vi "Gunsim Simulate.vi"(1 "Robot Constants":T4={"Distance from Pivot Point to Drive Mount(in)"=2.0, "Distance from Pivot Point to Arm Mount(in)"=2.0, "Distance from Pivot Point to Launcher(in)"=2.0, "Distance from Pivot Point to Camera(in)"=2.0, "WheelEncoder Ticks/Revolution"=2.0, "Wheel Radius"=2.0, "Triangle Angle(degrees)"=2.0, "Minimum LA Distance(inches)"=2.0, "LA Distance/Tick(inches)"=2.0}, 2 "cluster in":T3, 3 "Other Constants":T2={"Ball Diameter(in)"=10.0, "Air Density(g/in^3)"=0.02, "Drag coefficient"=0.5, "Ball Mass(g)"=300.0, "gravity(in/s^2)"=-386.09, "Minimum Goal Height(in)"=90.0, "Maximum Goal Height(in)"=104.0}, 4 "Parameters":T1) -> (0 "Range":T5)   [LabVIEW 2015]
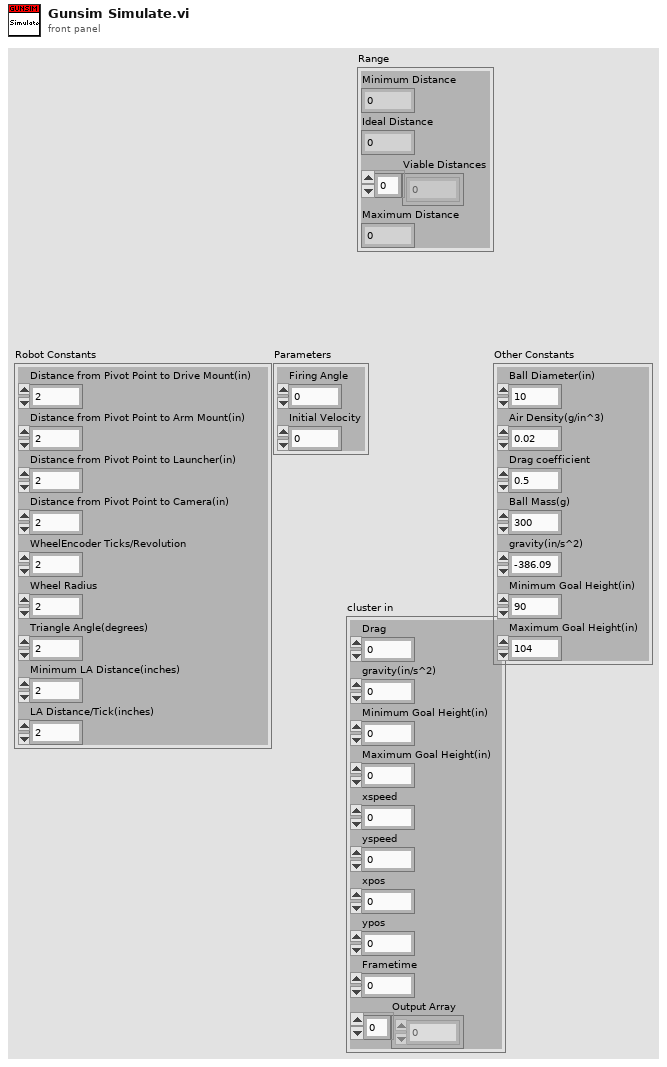
[diagram p1: front panel]
types:
  T1 = cluster{"Firing Angle":dbl, "Initial Velocity":dbl}
  T2 = cluster{"Ball Diameter(in)":dbl, "Air Density(g/in^3)":dbl, "Drag coefficient":dbl, "Ball Mass(g)":dbl, "gravity(in/s^2)":dbl, "Minimum Goal Height(in)":dbl, "Maximum Goal Height(in)":dbl}
  T3 = cluster{"Drag":dbl, "gravity(in/s^2)":dbl, "Minimum Goal Height(in)":dbl, "Maximum Goal Height(in)":dbl, "xspeed":dbl, "yspeed":dbl, "xpos":dbl, "ypos":dbl, "Frametime":dbl, "Output Array":dbl[]}
  T4 = cluster{"Distance from Pivot Point to Drive Mount(in)":dbl, "Distance from Pivot Point to Arm Mount(in)":dbl, "Distance from Pivot Point to Launcher(in)":dbl, "Distance from Pivot Point to Camera(in)":dbl, "WheelEncoder Ticks/Revolution":dbl, "Wheel Radius":dbl, "Triangle Angle(degrees)":dbl, "Minimum LA Distance(inches)":dbl, "LA Distance/Tick(inches)":dbl}
  T5 = cluster{"Minimum Distance":dbl, "Ideal Distance":dbl, "Viable Distances":dbl[], "Maximum Distance":dbl}
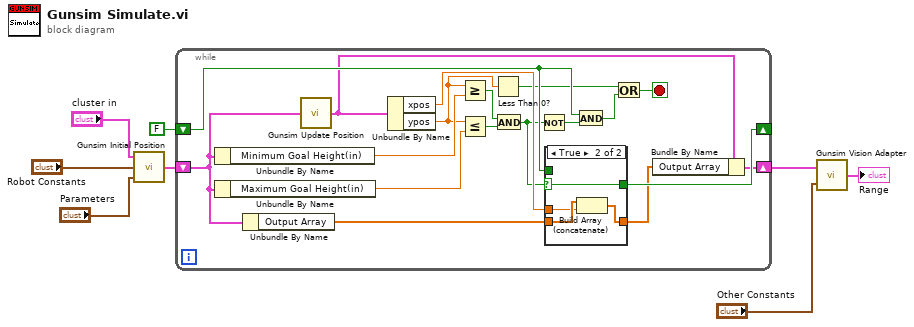
[diagram p0: block diagram]
diagram:
  n1 = call "Gunsim Initial Position.vi"("Parameters"="Parameters", "Robot Constants"="Robot Constants", "cluster in"="cluster in") -> ("cluster out"=w5:T3)
  n2 = while {
    shift-right: [w20] -> _
    shift-left: FALSE -> [w19]
    shift-right: [w9] -> w6
    shift-left: w5 -> [w13]
    stop <- w14 stop-if-true
    n3 = Unbundle By Name(w13) -> ("Minimum Goal Height(in)"=w23:dbl)
    n4 = Unbundle By Name(w13) -> ("Maximum Goal Height(in)"=w24:dbl)
    n5 = Unbundle By Name(w13) -> ("Output Array"=w12:dbl[])
    n6 = call "Gunsim Update Position.vi"("cluster in"=w13) -> ("cluster out"=w11:T3)
    n7 = Unbundle By Name(w11) -> ("xpos"=w22:dbl, "ypos"=w16:dbl)
    n8 = Greater Or Equal?(x=w16, y=w23) -> (x >= y?=w26:bool)
    n9 = Less Or Equal?(x=w16, y=w24) -> (x <= y?=w25:bool)
    n10 = Less Than 0?(x=w16) -> (x < 0?=w17:bool)
    n11 = And(x=w26, y=w25) -> (x .and. y?=w18:bool)
    n12 = Not(x=w18) -> (.not. x?=w21:bool)
    n13 = case shown="True" w18 {
      selector: w18 -> [_ w32]
      tunnel: w22 -> [_ w30]
      tunnel: w12 -> [w28 w31]
      tunnel: [w28 w29] -> w10
      tunnel: [w27 w32] -> w20
      tunnel: w19 -> [w27 _]
      frame False {
      }
      frame True {
        n14 = Build Array (concatenate)(w31, w30) -> (w29:dbl[])
      }
    }
    n15 = And(x=w19, y=w21) -> (x .and. y?=w15:bool)
    n16 = Or(x=w17, y=w15) -> (x .or. y?=w14:bool)
    n17 = Bundle By Name(cluster=w11, "Output Array"=w10) -> (w9:T3)
  }
  n18 = call "Gunsim Vision Adapter.vi"("Other Constants"="Other Constants", "cluster in"=w6) -> ("cluster out"=→"Range":T5)
